vi "init and update listboxes.vi"(8 "error in (no error)":errorcluster, 9 "table":refnum<vi>, 10 "display":refnum<vi>) -> (0 "error out":errorcluster, 2 "selected values":bool[](array[boolean]))   [LabVIEW 2016, in "FPGA RM System Definition API.lvlib"]
uses:
  FPGA-Resource-Manager-APIs/Source/System Definition/FPGA RM System Definition API.lvlib
  visualizer globals.vi
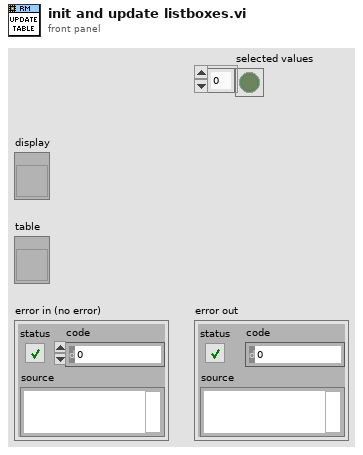
[diagram p1: front panel]
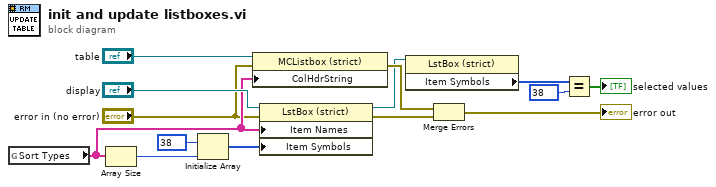
[diagram p0: block diagram]
diagram:
  n1 = global read "visualizer globals.vi" "Sort Types"() -> (w9:string[])
  n2 = Array Size(array=w9) -> (size(s)=w11:i32)
  n3 = Initialize Array(38, w11) -> (w10:i32[])
  n4 = property class="MCListbox (strict)"(reference="table", error in="error in (no error)", "ColHdrString"=w9) -> (error out=w6:errorcluster)  [unwired: 1 out]
  n5 = property on="Property Node" class="LstBox (strict)"(reference="display", error in="error in (no error)", "Item Names"=w9, "Item Symbols"=w10) -> (reference out=w4:refnum<vi>, error out=w14:errorcluster)
  n6 = property class="LstBox (strict)"(reference=w4) -> ("Item Symbols"=w2:i32[])  [unwired: 1 in, 2 out]
  n7 = Merge Errors(w6, w14) -> (→"error out":errorcluster)
  n8 = Equal?(x=w2, y=38) -> (x = y?=→"selected values":bool[])
